vi "Create.vi"(0 "ClassWriterNative":refnum<class "ClassWriterNative.lvclass">, 5 "error in (no error)":errorcluster) -> (14 "ClassWriterNative":refnum<class "ClassWriterNative.lvclass">, 19 "error out":errorcluster)   [LabVIEW 2020, in "ClassWriterNative.lvclass"]
doc: "Creates and initializes a new ClassWriterNative object.\n\nThis object should be destroyed using a ClassWriterNative destructor VI or a virtual base class destructor VI.\n\n[GOOP 2.0.16]"
uses:
  <resource>/Framework/Providers/Open_GDS/ClassProviders/Provider_LvNativeClass/ClassWriterNative_class/ClassWriterNative.lvclass
  <resource>/Framework/Providers/Open_GDS/ClassProviders/Provider_BaseClassInterface/ClassWriter_class/ClassWriter.lvclass
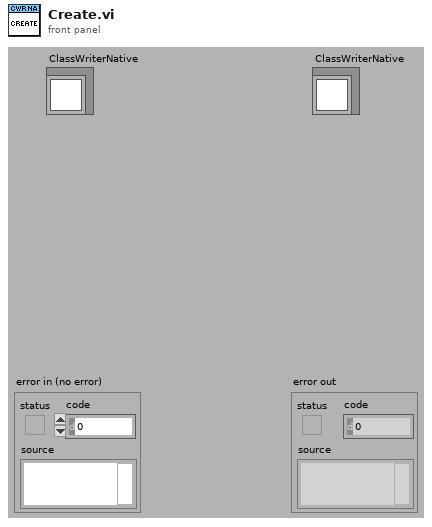
[diagram p1: front panel]
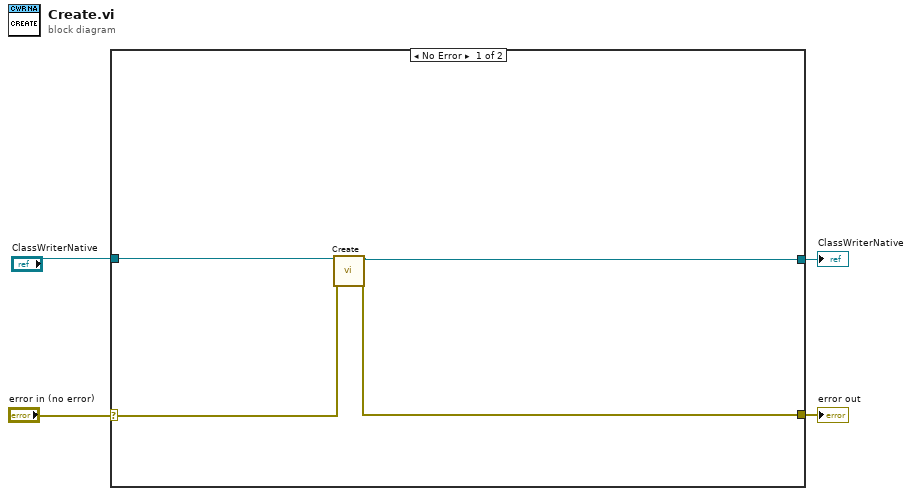
[diagram p0: block diagram]
diagram:
  n1 = case shown="No Error" "error in (no error)" {
    selector: "error in (no error)" -> [w7 w10]
    tunnel: [w5 w9] -> w4
    tunnel: [w6 w10] -> w3
    tunnel: "ClassWriterNative" -> [w8 w9]
    frame No Error {
      n2 = call-parent "Create.vi"("ClassWriter"=w8, "error in (no error)"=w7) -> ("ClassWriter"=w5:refnum<class "ClassWriterNative.lvclass">, "error out"=w6:errorcluster)  [unwired: 16 in]
    }
    frame Error {
    }
  }
  "error out" <- w3
  "ClassWriterNative" <- w4
